vi "mtg reader - read and display file.vi"(6 "max index":i32, 8 "index":i32, 9 "session file":string[][](table), 10 "data (sessions folder)":path, 11 "WaveformChart in":refnum<vi>) -> (2 "data (sessions folder) out":path, 3 "number of rows":i32)   [LabVIEW 2025]
uses:
  mtg reader - globals.vi
  <vilib>/Utility/file.llb/Read Delimited Spreadsheet (DBL).vi
panel:
  out "situation":u32
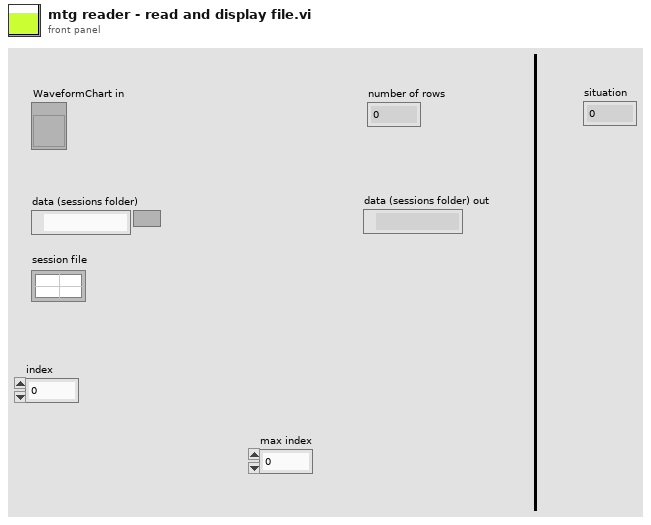
[diagram p1: front panel]
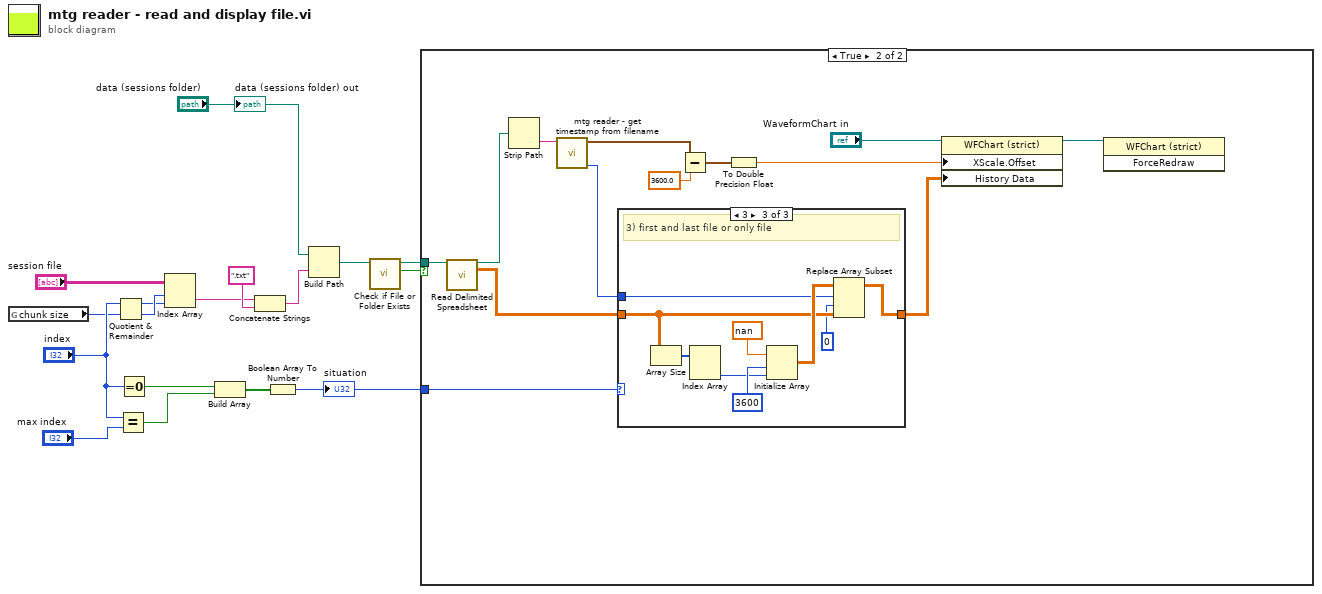
[diagram p0: block diagram]
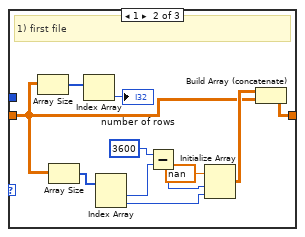
[diagram p4: hidden frame]
diagram:
  n1 = global read "mtg reader - globals.vi" "chunk size"() -> (w4:i32)
  n2 = Quotient & Remainder(x="index", y=w4) -> (x-y*floor(x/y)=w7:i32, floor(x/y)=w8:i32)
  n3 = Equal?(x="index", y="max index") -> (x = y?=w12:bool)
  n4 = Equal To 0?(x="index") -> (x = 0?=w13:bool)
  n5 = Index Array(array="session file", index (row)=w8, index (col)=w7) -> (element=w6:string)
  n6 = Build Array(w13, w12) -> (w11:bool[])
  n7 = Concatenate Strings(w6, ".txt" ("string")) -> (w16:string)
  n8 = Boolean Array To Number(Boolean array=w11) -> (number=w10:u32)
  "situation" <- w10
  n9 = Build Path(base path="data (sessions folder)", name or relative path=w16) -> (appended path=w3:path)
  n10 = call <vilib>:"Check if File or Folder Exists.vi"("path"=w3) -> ("file or folder exists?"=w1:bool, "dup path"=w2:path)  [unwired: 8 in, 1 out]
  n11 = case shown="True" w1 {
    tunnel: w10 -> [_ w22]
    tunnel: w2 -> [_ w18]
    frame False {
    }
    frame True {
      n12 = call-poly <vilib>:"Read Delimited Spreadsheet.vi"("file path (dialog if empty)"=w18) -> ("new file path (Not A Path if cancelled)"=w24:path, "all rows"=w23:dbl[][])  [unwired: 9 in, 4 out]
      n13 = Strip Path(path=w24) -> (name=w25:string)  [unwired: 1 out]
      n14 = call "mtg reader - get timestamp from filename.vi"("name"=w25) -> ("offset"=w20:i32, "Time Stamp"=w26:timestamp)  [unwired: 8 in, 1 out]
      n15 = case shown="3" w22 {
        tunnel: w23 -> [w31 w33 w46]
        tunnel: [w31 w32 w47] -> w21
        tunnel: w20 -> [_ _ w44]
        frame 0, 2, Default {
          # "0) neither first nor last 2) last file"
        }
        frame 1 {
          # "1) first file"
          n16 = Array Size(array=w33) -> (size(s)=w42:i32[])
          n17 = Array Size(array=w33) -> (size(s)=w39:i32[])
          n18 = Index Array(array=w42) -> (element=→"number of rows":i32)  [unwired: 1 in]
          n19 = Index Array(array=w39) -> (element #1=w36:i32, element #2=w38:i32)  [unwired: 2 in]
          n20 = Subtract(x=3600 ("dimension size"), y=w36) -> (x-y=w35:i32)
          n21 = Initialize Array(nan ("element"), w35, w38) -> (w34:dbl[][])
          n22 = Build Array (concatenate)(w34, w33) -> (w32:dbl[][])
        }
        frame 3 {
          # "3) first and last file or only file"
          n23 = Array Size(array=w46) -> (size(s)=w51:i32[])
          n24 = Index Array(array=w51) -> (element #2=w45:i32)  [unwired: 2 in, 1 out]
          n25 = Initialize Array(nan, 3600 ("dimension size"), w45) -> (w48:dbl[][])
          n26 = Replace Array Subset(array=w48, new element=w46, index (row)=w44, index (col)=0 ("disabled index (col)")) -> (w47:dbl[][])
        }
      }
      n27 = Subtract(x=w26, y=3600.0) -> (x-y=w28:timestamp)
      n28 = To Double Precision Float(number=w28) -> (double precision float=w30:dbl)
      n29 = property class="WFChart (strict)"(reference="WaveformChart in", "XScale.Offset"=w30, "History Data"=w21) -> (reference out=w19:refnum<vi>)  [unwired: 1 in, 1 out]
      n30 = invoke class="WFChart (strict)" method="ForceRedraw"(reference=w19) -> ()  [unwired: 2 in, 3 out]
    }
  }
  "data (sessions folder) out" <- "data (sessions folder)"
